vi "Font Color.vi"(8 "error in (no error)":errorcluster, 11 "Folder Item in":refnum<class "Folder Item.lvclass">) -> (0 "error out":errorcluster, 2 "Font Color":u32(colorbox), 3 "Folder Item out":refnum<class "Folder Item.lvclass">)   [LabVIEW 2020, in "BetterDragAndDropDemo.lvlib" / "Folder Item.lvclass"]
uses:
  Folder Item.lvclass
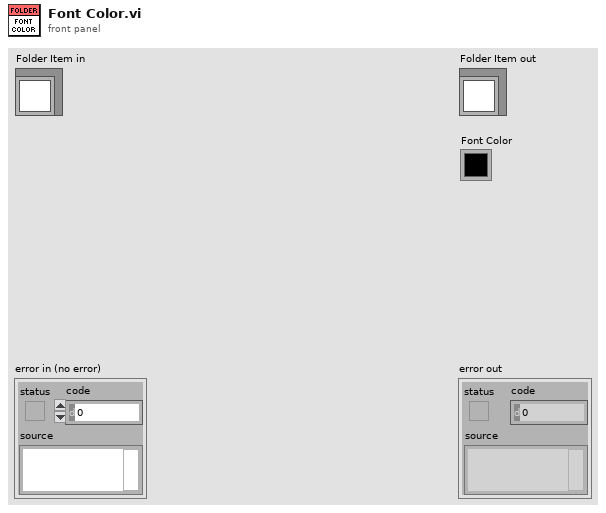
[diagram p1: front panel]
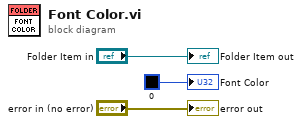
[diagram p0: block diagram]
diagram:
  "error out" <- "error in (no error)"
  "Folder Item out" <- "Folder Item in"
  "Font Color" <- u32 0
